vi "CoordinatesToPointer.vi"(8 "Input Type":T1(ring), 9 "Chunk length":u8, 10 "Voxel length":dbl, 11 "Coordinates":cluster{dbl, dbl, dbl}) -> (3 "Voxel pointer":cluster{i32, i32, i32, i32, i32, i32, i32})   [LabVIEW 2014]
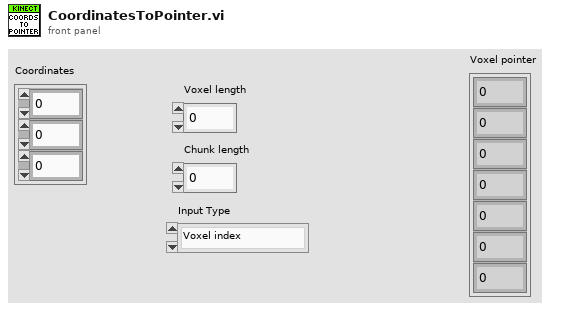
[diagram p1: front panel]
types:
  T1 = enum16{"Voxel index", "Inches", "Voxel center (in)"}
  T2 = cluster{"Quadrant":i32, i32, i32, i32, i32, i32, i32}
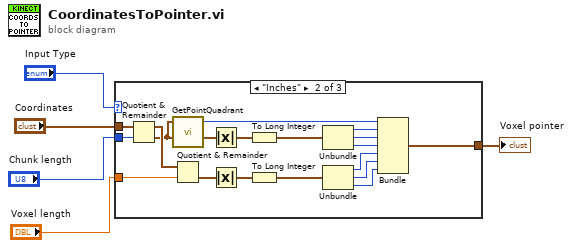
[diagram p0: block diagram]
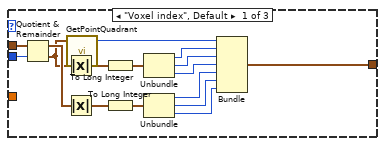
[diagram p2: hidden frame]
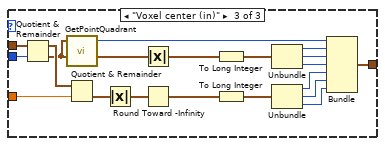
[diagram p3: hidden frame]
diagram:
  n1 = case shown="\"Inches\"" "Input Type" {
    tunnel: "Coordinates" -> [w20 w39 w58]
    tunnel: "Chunk length" -> [w21 w38 w57]
    tunnel: "Voxel length" -> [_ w36 w55]
    tunnel: [w6 w22 w42] -> w1
    frame "Voxel index", Default {
      n2 = Quotient & Remainder(x=w20, y=w21) -> (x-y*floor(x/y)=w19:cluster{dbl, dbl, dbl}, floor(x/y)=w18:cluster{dbl, dbl, dbl})
      n3 = Absolute Value(x=w18) -> (abs(x)=w16:cluster{dbl, dbl, dbl})
      n4 = Absolute Value(x=w19) -> (abs(x)=w10:cluster{dbl, dbl, dbl})
      n5 = call "GetPointQuadrant.vi"("Point"=w18) -> ("Quadrant"=w17:i32)  [unwired: 4 in]
      n6 = To Long Integer(number=w16) -> (32bit integer=w15:cluster{i32, i32, i32})
      n7 = To Long Integer(number=w10) -> (32bit integer=w9:cluster{i32, i32, i32})
      n8 = Unbundle(w15) -> (w14:i32, w13:i32, w12:i32)
      n9 = Unbundle(w9) -> (w11:i32, w8:i32, w7:i32)
      n10 = Bundle("Quadrant"=w17, w14, w13, w12, w11, w8, w7) -> (w6:T2)  [unwired: 1 in]
    }
    frame "Inches" {
      n11 = Quotient & Remainder(x=w39, y=w38) -> (x-y*floor(x/y)=w37:cluster{dbl, dbl, dbl}, floor(x/y)=w35:cluster{dbl, dbl, dbl})
      n12 = call "GetPointQuadrant.vi"("Point"=w35) -> ("Quadrant"=w31:i32)  [unwired: 4 in]
      n13 = Quotient & Remainder(x=w37, y=w36) -> (floor(x/y)=w34:cluster{dbl, dbl, dbl})  [unwired: 1 out]
      n14 = Absolute Value(x=w35) -> (abs(x)=w33:cluster{dbl, dbl, dbl})
      n15 = Absolute Value(x=w34) -> (abs(x)=w32:cluster{dbl, dbl, dbl})
      n16 = To Long Integer(number=w33) -> (32bit integer=w30:cluster{i32, i32, i32})
      n17 = To Long Integer(number=w32) -> (32bit integer=w29:cluster{i32, i32, i32})
      n18 = Unbundle(w30) -> (w28:i32, w27:i32, w26:i32)
      n19 = Unbundle(w29) -> (w25:i32, w24:i32, w23:i32)
      n20 = Bundle("Quadrant"=w31, w28, w27, w26, w25, w24, w23) -> (w22:T2)  [unwired: 1 in]
    }
    frame "Voxel center (in)" {
      n21 = Quotient & Remainder(x=w58, y=w57) -> (x-y*floor(x/y)=w56:cluster{dbl, dbl, dbl}, floor(x/y)=w54:cluster{dbl, dbl, dbl})
      n22 = call "GetPointQuadrant.vi"("Point"=w54) -> ("Quadrant"=w50:i32)  [unwired: 4 in]
      n23 = Quotient & Remainder(x=w56, y=w55) -> (floor(x/y)=w53:cluster{dbl, dbl, dbl})  [unwired: 1 out]
      n24 = Absolute Value(x=w53) -> (abs(x)=w51:cluster{dbl, dbl, dbl})
      n25 = Absolute Value(x=w54) -> (abs(x)=w52:cluster{dbl, dbl, dbl})
      n26 = Round Toward -Infinity(1:w51) -> (0:w41:cluster{dbl, dbl, dbl})
      n27 = To Long Integer(number=w52) -> (32bit integer=w49:cluster{i32, i32, i32})
      n28 = To Long Integer(number=w41) -> (32bit integer=w40:cluster{i32, i32, i32})
      n29 = Unbundle(w49) -> (w48:i32, w47:i32, w46:i32)
      n30 = Unbundle(w40) -> (w45:i32, w44:i32, w43:i32)
      n31 = Bundle("Quadrant"=w50, w48, w47, w46, w45, w44, w43) -> (w42:T2)  [unwired: 1 in]
    }
  }
  "Voxel pointer" <- w1
